vi "update.properties.request.vi"(8 "error in":errorcluster, 11 "properties":map{string, string}(c390)) -> (0 "error out":errorcluster, 1 "Request":string)   [LabVIEW 2020, in "Run.lvclass"]
uses:
  <vilib>/JDP Science/JSONtext/support/Format JSON Object.vi
  Run.lvclass
  Run.lvclass/Run.ctl
  <vilib>/JDP Science/JSONtext/JSONtext.lvlib
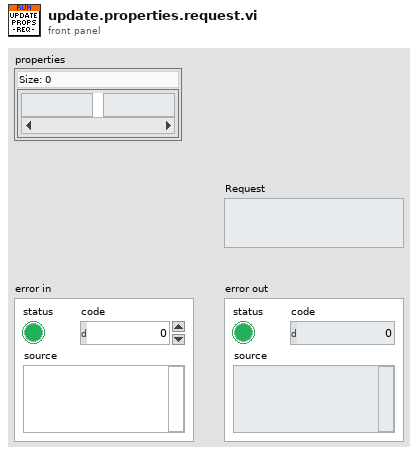
[diagram p1: front panel]
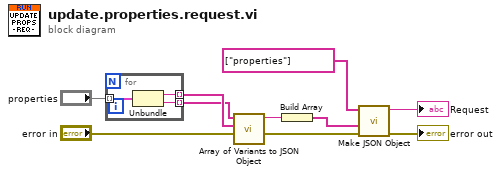
[diagram p0: block diagram]
diagram:
  n1 = for {
    tunnel: "properties" -> [w13] mode=indexing
    tunnel: [w12] -> w9 mode=indexing
    tunnel: [w11] -> w8 mode=indexing
    n2 = Unbundle(w13) -> ("name"=w12:string, "value"=w11:string)
  }
  n3 = call <vilib>:"Array of Variants to JSON Object.vi"("error in (no error)"="error in", "Names"=w9, "Array"=w8) -> ("error out"=w4:errorcluster, "<JSON>"=w6:string)  [unwired: 7 in]
  n4 = Build Array(w6) -> (w5:string[])
  n5 = call <vilib>:"Make JSON Object.vi"("error in (no error)"=w4, "JSON Items"=w5, "Item Names"=string[] ["properties"]) -> ("error out"=→"error out":errorcluster, "<JSON>"=→"Request":string)  [unwired: 7 in]
